vi "CF_FP_to_DSC.vi"(0 "str":string[](array[string]), 1 "str var":refnum<k21>[](array[refnum])=["ni.var.psp://housesoftheholy/Leiden CF900/CF_FP_STATE"], 2 "dbl":dbl[](array[numeric]), 3 "dbl var":refnum<k21>[](array[refnum])=["ni.var.psp://housesoftheholy/Leiden CF900/Leiden CF FP/CF FP P1", "ni.var.psp://housesoftheholy/Leiden CF900/Leiden CF FP/CF FP P2", "ni.var.psp://housesoftheholy/Leiden CF900/Leiden CF FP/CF FP P3", "ni.var.psp://housesoftheholy/Leiden CF900/Leiden CF FP/CF FP P4", "ni.var.psp://housesoftheholy/Leiden CF900/Leiden CF FP/CF FP P5", "ni.var.psp://housesoftheholy/Leiden CF900/Leiden CF FP/CF FP P6", "ni.var.psp://housesoftheholy/Leiden CF900/Leiden CF FP/CF FP P7", "ni.var.psp://housesoftheholy/Leiden CF900/Leiden CF FP/CF FP Flow", "ni.var.psp://housesoftheholy/Leiden CF900/Leiden CF FP/CF FP MG0", "ni.var.psp://housesoftheholy/Leiden CF900/Leiden CF FP/CF FP MG1", "ni.var.psp://housesoftheholy/Leiden CF900/Leiden CF FP/CF FP MG2", "ni.var.psp://housesoftheholy/Leiden CF900/Leiden CF FP/CF FP MG3", "ni.var.psp://housesoftheholy/Leiden CF900/Leiden CF FP/CF FP MG4", "ni.var.psp://housesoftheholy/Leiden CF900/Leiden CF FP/CF FP MG5", "ni.var.psp://housesoftheholy/Leiden CF900/Leiden CF FP/CF FP PT on", "ni.var.psp://housesoftheholy/Leiden CF900/Leiden CF FP/CF FP W_in", "ni.var.psp://housesoftheholy/Leiden CF900/Leiden CF FP/CF FP W_out", "ni.var.psp://housesoftheholy/Leiden CF900/Leiden CF FP/CF FP He", "ni.var.psp://housesoftheholy/Leiden CF900/Leiden CF FP/CF FP oil", "ni.var.psp://housesoftheholy/Leiden CF900/Leiden CF FP/CF FP P_low", "ni.var.psp://housesoftheholy/Leiden CF900/Leiden CF FP/CF FP P_high", "ni.var.psp://housesoftheholy/Leiden CF900/Leiden CF FP/CF FP PT current", "ni.var.psp://housesoftheholy/Leiden CF900/Leiden CF FP/CF FP state0", "ni.var.psp://housesoftheholy/Leiden CF900/Leiden CF FP/CF FP state1", "ni.var.psp://housesoftheholy/Leiden CF900/Leiden CF FP/CF FP state2"]) -> ()   [LabVIEW 2013]
panel:
  # "CF FP to DSC"
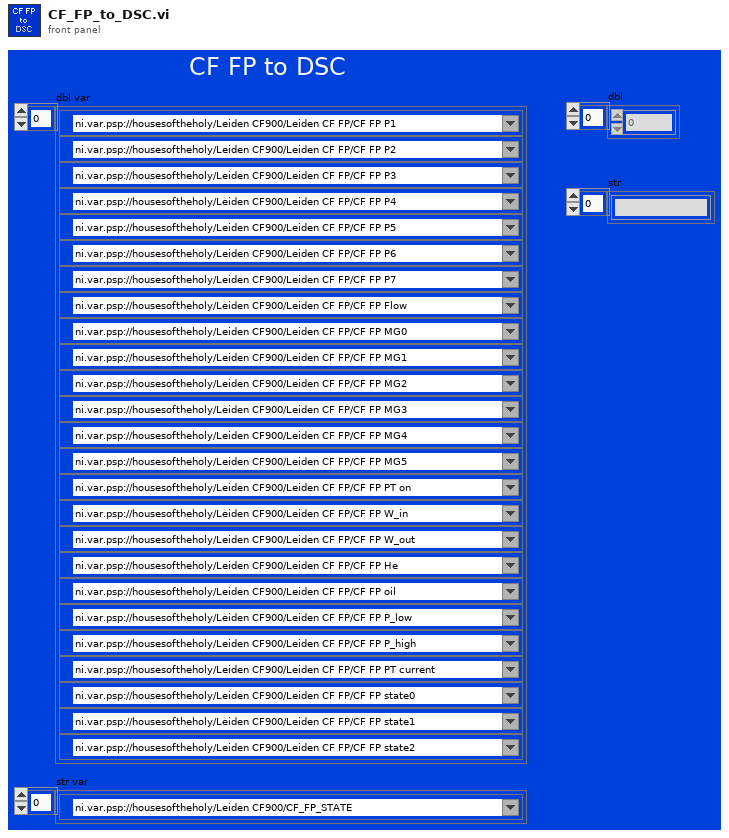
[diagram p1: front panel]
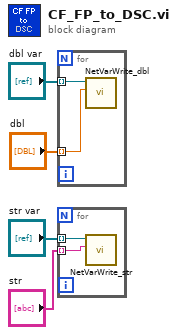
[diagram p0: block diagram]
diagram:
  n1 = for {
    tunnel: "dbl var" -> [w6] mode=indexing
    tunnel: "dbl" -> [w5] mode=indexing
    n2 = call "NetVarWrite_dbl.vi"("Numeric"=w5, "Refnum in"=w6) -> ()  [unwired: 10 in]
  }
  n3 = for {
    tunnel: "str var" -> [w8] mode=indexing
    tunnel: "str" -> [w7] mode=indexing
    n4 = call "NetVarWrite_str.vi"("String"=w7, "Refnum in"=w8) -> ()  [unwired: 10 in]
  }
